vi "PT Settings Dialog.vi"(8 "error in (no error)":errorcluster, 11 "PT Module Config in":T2) -> (0 "error out":errorcluster, 1 "Cancelled?":bool=TRUE, 2 "UI Refresh Needed?":bool, 3 "PT Module Config out":T2)   [LabVIEW 2018, in "PT Module.lvlib"]
doc: "Dialog for selecting user specified settings."
uses:
  PT Module.lvlib
  Controls/PT Module Config Cluster.ctl
  <vilib>/Utility/miscctls.llb/LVPoint32TypeDef.ctl
  Controls/PT Settings Dialog.ctl
  Tag VIs/Tag FGV Operation Enum.ctl
  Shared Variables/Simple Alarm Values Cluster.ctl
  Shared Variables/Dynamic Shared Variables.lvlib
panel:
  in  "Module Name":string
  in  "Settings Dialog":T1 {"Input Channel Tag Name" items=["Temperature", "Temperature_0"]}
  in  "Cancel Button":bool
  in  "OK Button":bool
  # "Non visible portion of dialog (needed for connector pane)."
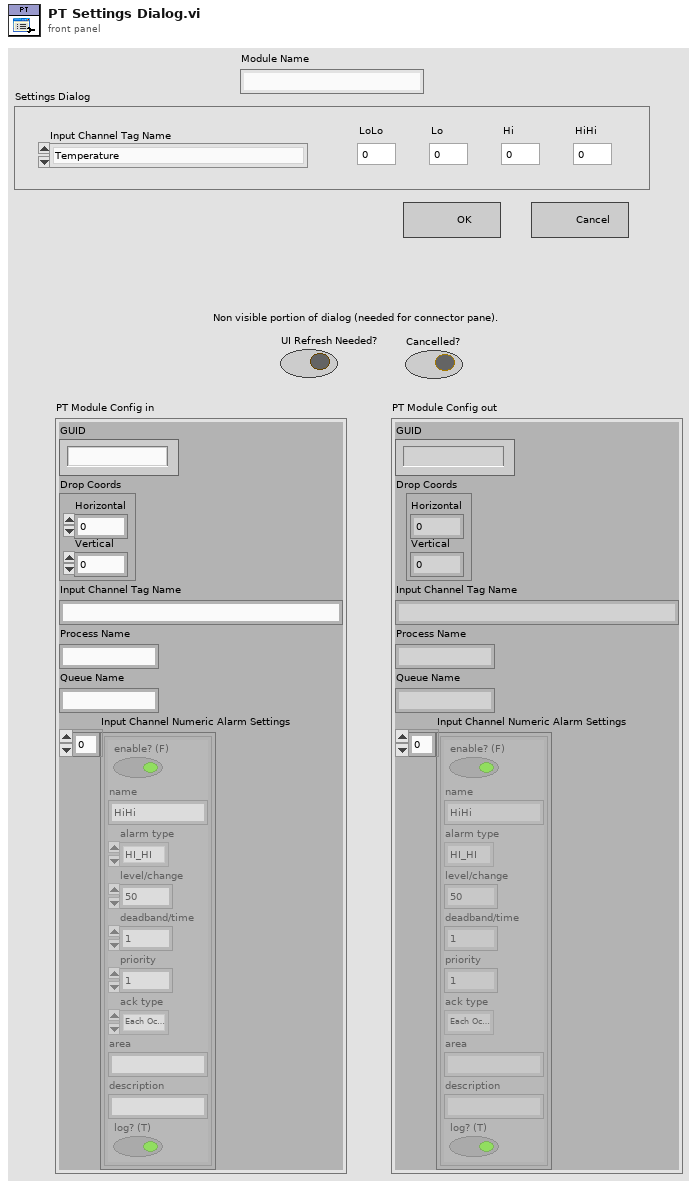
[diagram p1: front panel]
types:
  T1 = typedef "PT Module.lvlib/PT Settings Dialog.ctl" = cluster{"Input Channel Tag Name":u16, "LoLo":dbl, "Lo":dbl, "Hi":dbl, "HiHi":dbl}
  T2 = typedef "PT Module.lvlib/PT Module Config Cluster.ctl" = cluster{"GUID":string, "Drop Coords":T3, "Input Channel Tag Name ":string, "Process Name":string, "Queue Name":string, "Input Channel Numeric Alarm Settings":cluster{"enable? (F)":bool, "name":string, "alarm type":enum16{"HI_HI", "HI", "LO", "LO_LO"}, "level/change":dbl, "deadband/time":dbl, "priority":u32, "ack type":enum16{"Auto", "User", "None", "Each Occurrence"}, "area":string, "description":string, "log? (T)":bool}[]}
  T3 = typedef "LVPoint32TypeDef.ctl" = cluster{"Horizontal":i32, "Vertical":i32}
  T4 = typedef "Tag FGV Operation Enum.ctl" = enum16{"Init", "Set Notification Queue", "Create Tag", "Commit", "Write Tag (Numeric)", "Write Tag (Boolean)", "Read All Tags", "Read One Tag", "Delete Tag Category", "Set Alarm Parameters (Numeric)", "Set Alarm Parameters (Boolean)", "Enable All Alarms", "Disable All Alarms", "Delete All Tags", "Read Alarms", "Ack Alarm"}
  T5 = typedef "Dynamic Shared Variables.lvlib/Simple Alarm Values Cluster.ctl" = cluster{"tag name":string, "HiHi":dbl, "Hi":dbl, "Lo":dbl, "LoLo":dbl}
  T6 = cluster{"enable? (F)":bool, "name":string, "alarm type":enum16{"HI_HI", "HI", "LO", "LO_LO"}, "level/change":dbl, "deadband/time":dbl, "priority":u32, "ack type":enum16{"Auto", "User", "None", "Each Occurrence"}, "area":string, "description":string, "log? (T)":bool}[]
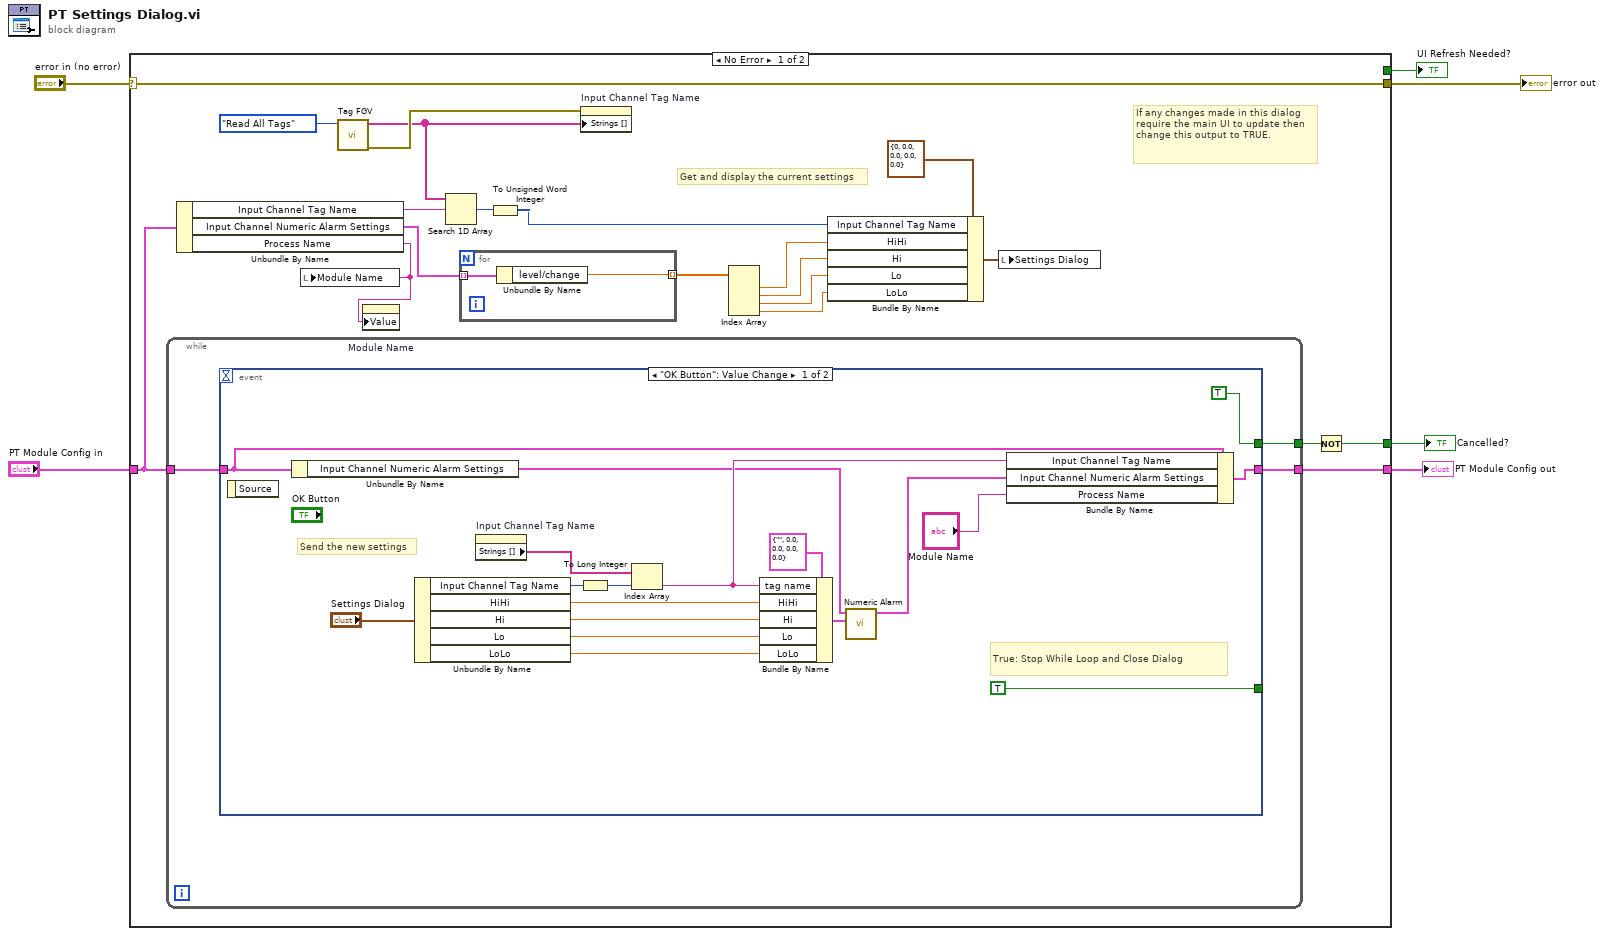
[diagram p0: block diagram]
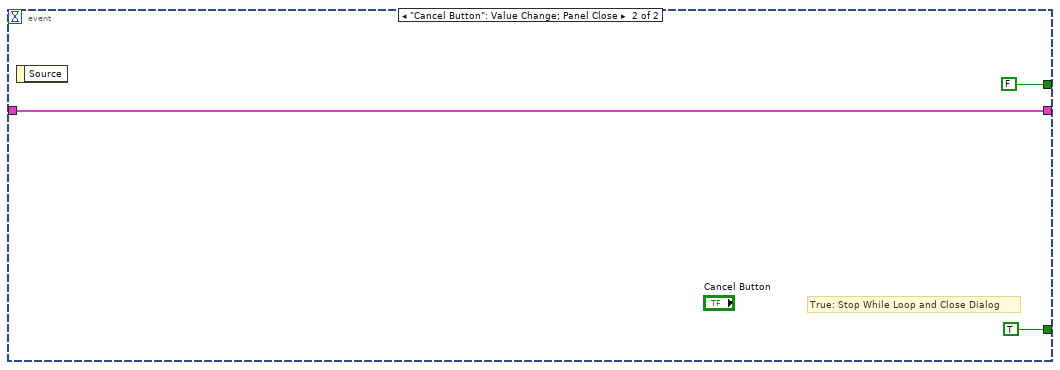
[diagram p2: hidden frame]
diagram:
  n1 = case shown="No Error" "error in (no error)" {
    selector: "error in (no error)" -> [w27 w57]
    tunnel: [w27 w57] -> w6
    tunnel: "PT Module Config in" -> [w24 w56]
    tunnel: [w25 w56] -> w1
    tunnel: [FALSE ("UI Refresh Needed?") _] -> w4
    tunnel: [w22 TRUE ("UI Refresh Needed?")] -> w3
    frame No Error {
      # "Get and display the current settings"
      # "If any changes made in this dialog require the main UI to update then change this output to TRUE."
      n2 = while {
        tunnel: [w33] -> w23
        tunnel: [w30] -> w25
        tunnel: w24 -> [w32]
        stop <- w31 stop-if-true
        n3 = event shown="[0] \"OK Button\": Value Change" {
          selector: _ -> [_ _]
          dyn-events: _ -> [_ _]
          timeout: _ -> [_ _]
          tunnel: w32 -> [w38 w54]
          tunnel: [TRUE ("UI Refresh Needed?") FALSE ("UI Refresh Needed?")] -> w33
          tunnel: [TRUE TRUE] -> w31
          tunnel: [w49 w54] -> w30
          event "OK Button": Value Change {
            # "Send the new settings"
            # "True: Stop While Loop and Close Dialog"
            n4 = event-data() -> ()  [unwired: 1 in, 1 out]
            n5 = Unbundle By Name(w38) -> ("Input Channel Numeric Alarm Settings"=w37:T6)
            n6 = Unbundle By Name("Settings Dialog") -> ("Input Channel Tag Name"=w47:u16, "HiHi"=w46:dbl, "Hi"=w45:dbl, "Lo"=w44:dbl, "LoLo"=w34:dbl)
            n7 = property on="Input Channel Tag Name" class="Ring (strict)"() -> ("Strings []"=w48:string[])  [unwired: 2 in, 2 out]
            n8 = To Long Integer(number=w47) -> (32bit integer=w41:i32)
            n9 = Index Array(array=w48, index=w41) -> (element=w40:string)
            n10 = Bundle By Name(cluster=T5 {"tag name"="", "HiHi"=0.0, "Hi"=0.0, "Lo"=0.0, "LoLo"=0.0} ("Simple Alarm Values"), "tag name"=w40, "HiHi"=w46, "Hi"=w45, "Lo"=w44, "LoLo"=w34) -> (w42:T5)
            n11 = call "Numeric Alarm.vi"("Simple Alarm Values"=w42, "Alarms in"=w37) -> ("Alarms out"=w36:T6)  [unwired: 9 in]
            n12 = Bundle By Name(cluster=w38, "Input Channel Tag Name"=w40, "Input Channel Numeric Alarm Settings"=w36, "Process Name"="Module Name") -> (w49:T2)
          }
          event "Cancel Button": Value Change; Panel Close {
            # "True: Stop While Loop and Close Dialog"
            n13 = event-data() -> ()  [unwired: 1 in, 1 out]
          }
        }
      }
      n14 = Unbundle By Name(w24) -> ("Input Channel Tag Name"=w18:string, "Input Channel Numeric Alarm Settings"=w10:T6, "Process Name"=w7:string)
      n15 = local write "Module Name"(w7) -> ()
      n16 = call "Tag FGV.vi"("Operation"=Tag_FGV_Operation_Enum."Read All Tags") -> ("error out"=w21:errorcluster, "Tag Names"=w19:string[])  [unwired: 5 in, 4 out]
      n17 = property on="Module Name" class="Str"("Value"=w7) -> ()  [unwired: 2 in, 2 out]
      n18 = Search 1D Array(1D array=w19, element=w18) -> (index of element=w17:i32)  [unwired: 1 in]
      n19 = for {
        tunnel: w10 -> [w29] mode=indexing
        tunnel: [w28] -> w9 mode=indexing
        n20 = Unbundle By Name(w29) -> ("level/change"=w28:dbl)
      }
      n21 = To Unsigned Word Integer(number=w17) -> (unsigned 16bit integer=w8:u16)
      n22 = property on="Input Channel Tag Name" class="Ring (strict)"(error in=w21, "Strings []"=w19) -> ()  [unwired: 1 in, 2 out]
      n23 = Index Array(array=w9) -> (element #1=w14:dbl, element #2=w13:dbl, element #3=w12:dbl, element #4=w11:dbl)  [unwired: 4 in]
      n24 = Bundle By Name(cluster=T1 {"Input Channel Tag Name"=0, "LoLo"=0.0, "Lo"=0.0, "Hi"=0.0, "HiHi"=0.0} ("Settings Dialog"), "Input Channel Tag Name"=w8, "HiHi"=w14, "Hi"=w13, "Lo"=w12, "LoLo"=w11) -> (w15:T1)
      n25 = local write "Settings Dialog"(w15) -> ()
      n26 = Not(x=w23) -> (.not. x?=w22:bool)
    }
    frame Error {
    }
  }
  "UI Refresh Needed?" <- w4
  "error out" <- w6
  "PT Module Config out" <- w1
  "Cancelled?" <- w3
